vi "ELAPSED TIMMER VI.vi"(3 "error in (no error)":errorcluster, 4 "TARGET VALUE":dbl, 5 "RESET":bool, 6 "PAUSE":bool) -> (0 "error IO":errorcluster, 1 "ELAPSED TIMMER":bool, 2 "ELAPSED TIMER VALUE":dbl)   [LabVIEW 2023]
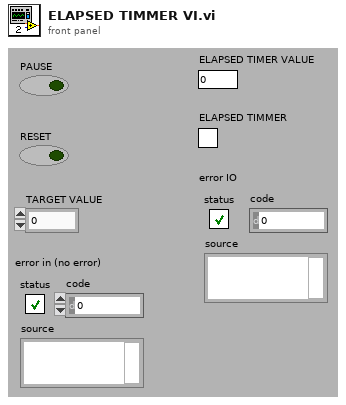
[diagram p1: front panel]
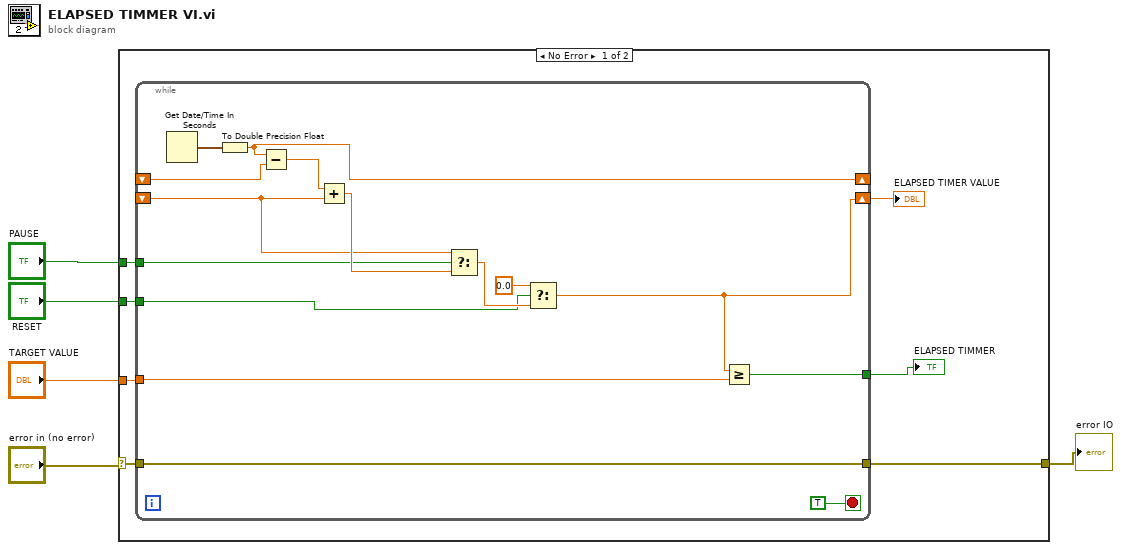
[diagram p0: block diagram]
diagram:
  n1 = case shown="No Error" "error in (no error)" {
    selector: "error in (no error)" -> [w6 _]
    tunnel: "PAUSE" -> [w10 _]
    tunnel: "RESET" -> [w9 _]
    tunnel: "TARGET VALUE" -> [w8 _]
    tunnel: [w7 _] -> w5
    frame No Error {
      n2 = while {
        shift-right: [w24] -> _
        shift-left: _ -> [w25]
        shift-right: [w19] -> w11
        shift-left: _ -> [w18]
        tunnel: [w17] -> w12
        tunnel: w10 -> [w16]
        tunnel: w9 -> [w15]
        tunnel: w8 -> [w14]
        tunnel: [w13] -> w7
        tunnel: w6 -> [w13]
        stop <- TRUE ("stop") stop-if-true
        n3 = Get Date/Time In Seconds() -> (seconds since 1Jan1904=w26:timestamp)
        n4 = To Double Precision Float(number=w26) -> (double precision float=w24:dbl)
        n5 = Subtract(x=w24, y=w25) -> (x-y=w23:dbl)
        n6 = Add(x=w23, y=w18) -> (x+y=w22:dbl)
        n7 = Select(t=w18, s=w16, f=w22) -> (s? t:f=w21:dbl)
        n8 = Select(t=0.0, s=w15, f=w21) -> (s? t:f=w19:dbl)
        n9 = Greater Or Equal?(x=w19, y=w14) -> (x >= y?=w17:bool)
      }
      "ELAPSED TIMMER" <- w12
      "ELAPSED TIMER VALUE" <- w11
    }
    frame Error {
    }
  }
  "error IO" <- w5
